vi "Write Version Number from Package.vi"(8 "Error In":errorcluster, 11 "Package Version":T1) -> (0 "Error Out":errorcluster)   [LabVIEW 2017, in "Scripts.lvlib"]
uses:
  Scripts.lvlib
  <vilib>/JKI/VIPM API/command-line/support/Version Info Cluster_vipm_api.ctl
  <vilib>/AppBuilder/AB_API_Simple/Build Specification Version.ctl
  <vilib>/AppBuilder/AB_API_Simple/Set Build Specification Version (path).vi
  <vilib>/AppBuilder/AB_API_Simple/NI_App_Builder_API.lvlib
  <vilib>/JKI/VIPM API/VIPM API_vipm_api.lvlib
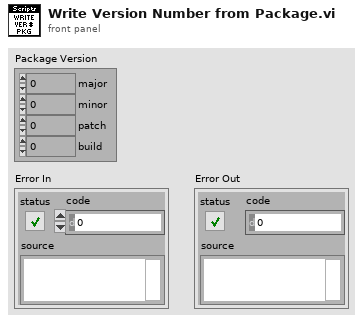
[diagram p1: front panel]
types:
  T1 = typedef "VIPM API_vipm_api.lvlib/Version Info Cluster_vipm_api.ctl" = cluster{"major":u32, "minor":u32, "patch":u32, "build":u32}
  T2 = typedef "NI_App_Builder_API.lvlib/Build Specification Version.ctl" = cluster{"Major":u16, "Minor":u16, "Fix":u16, "Build":u16}
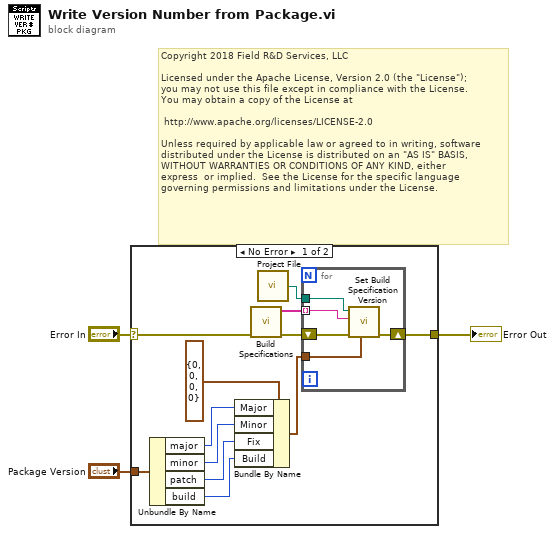
[diagram p0: block diagram]
diagram:
  # "Copyright 2018 Field R&D Services, LLC\n\nLicensed under the Apache License, Version 2.0 (the \"License\");\nyou may not use this file except in compliance with the License.\nYou may obtain a copy of the License at\n\n\thttp://www.apache.org/licenses/LICENSE-2.0\n\nUnless required by applicable law or agreed to in writing, software\ndistributed under the License is distributed on an \"AS IS\" BASIS,\nWITHOUT WARRANTIES OR CONDITIONS OF ANY KIND, either \nexpress  or implied.  See the License for the specific language \ngoverning permissions and limitations under the License."
  n1 = case shown="No Error" "Error In" {
    selector: "Error In" -> [w12 w21]
    tunnel: [w14 w21] -> w3
    tunnel: "Package Version" -> [w8 _]
    frame No Error {
      n2 = Unbundle By Name(w8) -> ("major"=w7:u32, "minor"=w6:u32, "patch"=w5:u32, "build"=w4:u32)
      n3 = Bundle By Name(cluster=T2 {"Major"=0, "Minor"=0, "Fix"=0, "Build"=0} ("Build Specification Version"), "Major"=w7, "Minor"=w6, "Fix"=w5, "Build"=w4) -> (w9:T2)
      n4 = call "Build Specifications.vi"("Error In"=w12) -> ("Error Out"=w11:errorcluster, "Build Specifications"=w15:string[])  [unwired: 9 in]
      n5 = call "Project File.vi"() -> ("Project File"=w13:path)
      n6 = for {
        tunnel: w13 -> [w20]
        shift-right: [w19] -> w14
        shift-left: w11 -> [w18]
        tunnel: w15 -> [w17] mode=indexing
        tunnel: w9 -> [w16]
        n7 = call-poly <vilib>:"Set Build Specification Version.vi"("Build Specification Version"=w16, "error in (no error)"=w18, "Name of build specification"=w17, "Path to project"=w20) -> ("error out"=w19:errorcluster)  [unwired: 7 in]
      }
    }
    frame Error {
    }
  }
  "Error Out" <- w3
